vi "Get_iniArry_KEY.vi"(8 "error in (no error)":errorcluster caption="错误输入（无错误）", 11 "section":string caption="段") -> (0 "error out":errorcluster, 2 "数组":string[](array[string]), 3 "key names":string[](array[string]) caption="键名")   [LabVIEW 2018]
uses:
  Global.vi
  <vilib>/Utility/config.llb/Read Key (String).vi
  <vilib>/Utility/config.llb/NI_LVConfig.lvlib
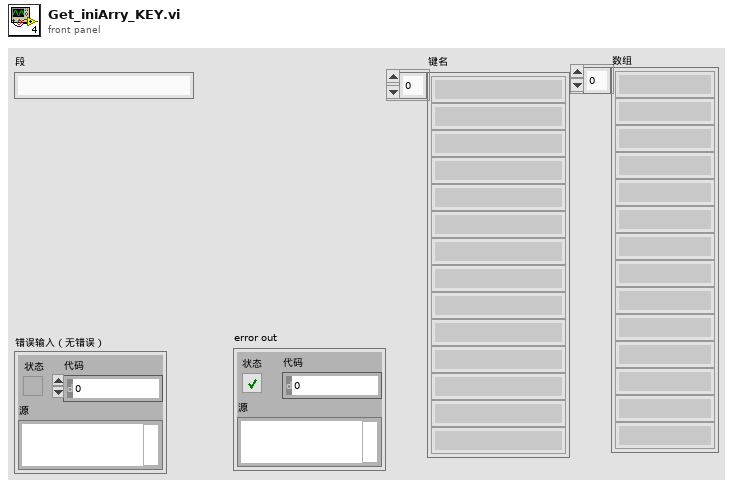
[diagram p1: front panel]
types:
  T1 = typedef "NI_LVConfig.lvlib/Config Data RefNum.ctl" = refnum<k1>
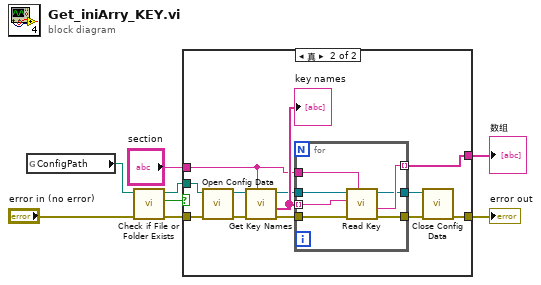
[diagram p0: block diagram]
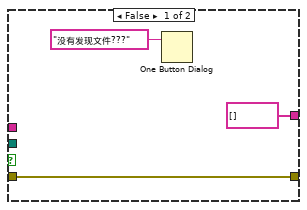
[diagram p2: hidden frame]
diagram:
  n1 = global read "Global.vi" "ConfigPath"() -> (w8:path)
  n2 = call <vilib>:"Check if File or Folder Exists.vi"("error in (no error)"="error in (no error)", "path"=w8) -> ("error out"=w3:errorcluster, "file or folder exists?"=w6:bool, "dup path"=w7:path)  [unwired: 7 in]
  n3 = case shown="真" w6 {
    tunnel: w7 -> [_ w23]
    tunnel: "section" -> [_ w19]
    tunnel: [string[] [] w17] -> w4
    tunnel: w3 -> [w9 w16]
    tunnel: [w9 w12] -> w2
    frame False {
      n4 = One Button Dialog(message="没有发现文件???" ("消息")) -> ()  [unwired: 1 in, 1 out]
    }
    frame True {
      n5 = call <vilib>:"Open Config Data.vi"("error in (no error)"=w16, "configuration file path"=w23) -> ("error out"=w22:errorcluster, "refnum"=w21:T1)  [unwired: 7 in, 1 out]
      n6 = call <vilib>:"Get Key Names.vi"("section"=w19, "error in (no error)"=w22, "refnum"=w21) -> ("error out"=w15:errorcluster, "key names"=w20:string[], "refnum out"=w18:T1)  [unwired: 5 in, 1 out]
      "key names" <- w20
      n7 = for {
        tunnel: w20 -> [w29] mode=indexing
        tunnel: w19 -> [w30]
        tunnel: [w28] -> w17 mode=indexing
        tunnel: w18 -> [w27]
        tunnel: w15 -> [w26]
        tunnel: [w25] -> w13
        tunnel: [w24] -> w14
        n8 = call-poly <vilib>:"Read Key.vi"("section"=w30, "error in (no error)"=w26, "key"=w29, "refnum"=w27) -> ("error out"=w25:errorcluster, "value"=w28:string, "refnum out"=w24:T1)  [unwired: 4 in, 1 out]
      }
      n9 = call <vilib>:"Close Config Data.vi"("error in (no error)"=w13, "refnum"=w14) -> ("error out"=w12:errorcluster)  [unwired: 8 in, 1 out]
    }
  }
  "数组" <- w4
  "error out" <- w2
